vi "LSX Get Dig Joy Speed.vi"(0 "lLSID":i32, 1 "pdR":dbl, 5 "pdX":dbl, 7 "pdY":dbl, 9 "pdZ":dbl, 11 "error in (no error)":errorcluster) -> (3 "pdR out":dbl, 4 "function return":i32, 6 "pdX out":dbl, 8 "pdY out":dbl, 10 "pdZ out":dbl, 15 "error out":errorcluster)   [LabVIEW 2016, in "Tango_DLL.lvlib"]
doc: "TANGOAPI int TANGOCALL LSX_GetDigJoySpeed (int lLSID, double *pdX, double *pdY, double *pdZ, double *pdR);"
uses:
  Tango_DLL.lvlib
  2017/Microscope Control/Device Library/Stages/Marzhauser/SCAN IM 120 x 80/Tango DLL VIs/Tango_DLL.dll
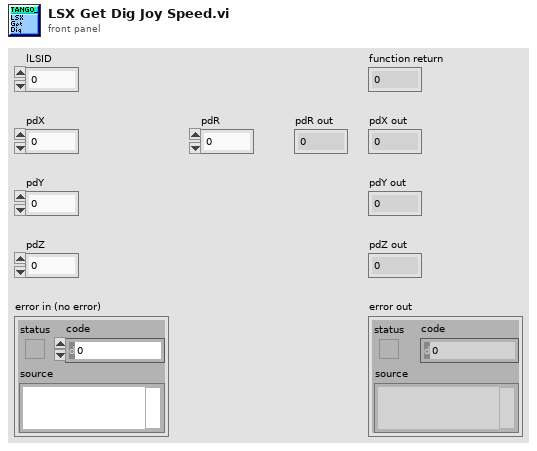
[diagram p1: front panel]
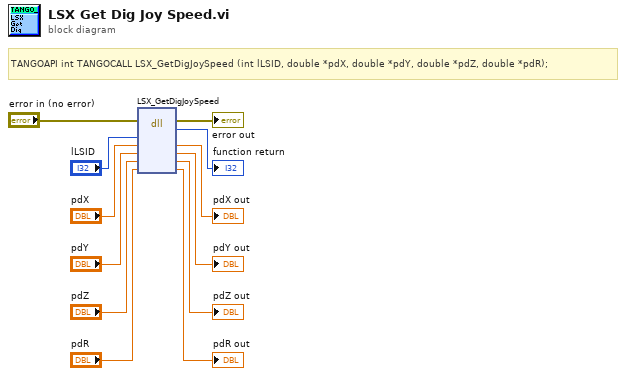
[diagram p0: block diagram]
diagram:
  # "TANGOAPI int TANGOCALL LSX_GetDigJoySpeed (int lLSID, double *pdX, double *pdY, double *pdZ, double *pdR);"
  n1 = dll-call lib="C:/Users/4PiSMS/Documents/Microscope Control/2017/Microscope Control/Device Library/Stages/Marzhauser/SCAN IM 120 x 80/Tango DLL VIs/Tango_DLL.*" fn="LSX_GetDigJoySpeed"(error in="error in (no error)", "lLSID"="lLSID", "pdX"="pdX", "pdY"="pdY", "pdZ"="pdZ", "pdR"="pdR") -> (error out=→"error out":errorcluster, →"function return":i32, "pdX"=→"pdX out":dbl, "pdY"=→"pdY out":dbl, "pdZ"=→"pdZ out":dbl, "pdR"=→"pdR out":dbl)  [unwired: 3 in, 1 out]
